vi "trig.vi"(8 "error in (no error)":errorcluster, 11 "p2p vst in":refnum<class "p2p vst.lvclass">) -> (0 "error out":errorcluster, 3 "p2p vst out":refnum<class "p2p vst.lvclass">)   [LabVIEW 2021, in "p2p vst.lvclass"]
uses:
  p2p vst.lvclass
  p2p vst.lvclass/p2p vst.ctl
  <instrlib>/niRFSG/niRFSG.llb/niRFSG Stream Endpoint Names.ctl
  <vilib>/FPGAPlugInAG/Dynamic/niLvFpga_P2PGetEndpoint_Dynamic.vi
  <vilib>/Utility/error.llb/Error Cluster From Error Code.vi
  <vilib>/rvi/errors/niLvFpgaAdjustHostInterfaceError.vi
  <vilib>/rvi/interface/nirviMethod/nirviMethod.xnode
  <vilib>/rvi/interface/nirviReadWriteControl/nirviReadWriteControl.xnode
  NiFpgaLv.dll
  <vilib>/rvi/interface/Simulation/niFpgaSimulationCallBeginRW.vi
  <vilib>/rvi/errors/niLvFpgaMergeErrorWithErrorCode.vi
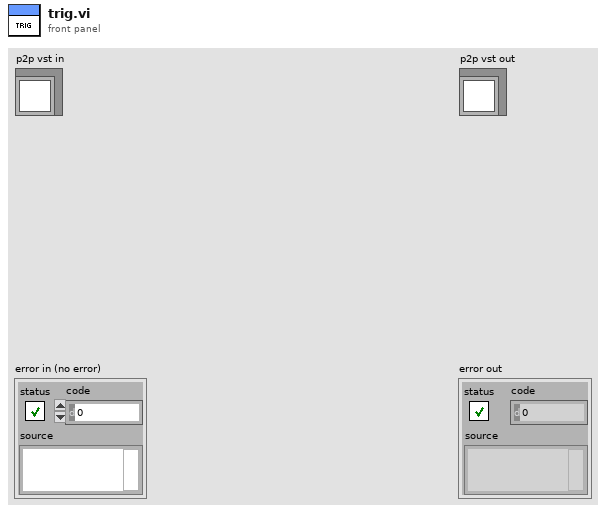
[diagram p1: front panel]
types:
  T1 = typedef "niRFSG Stream Endpoint Names.ctl" = string
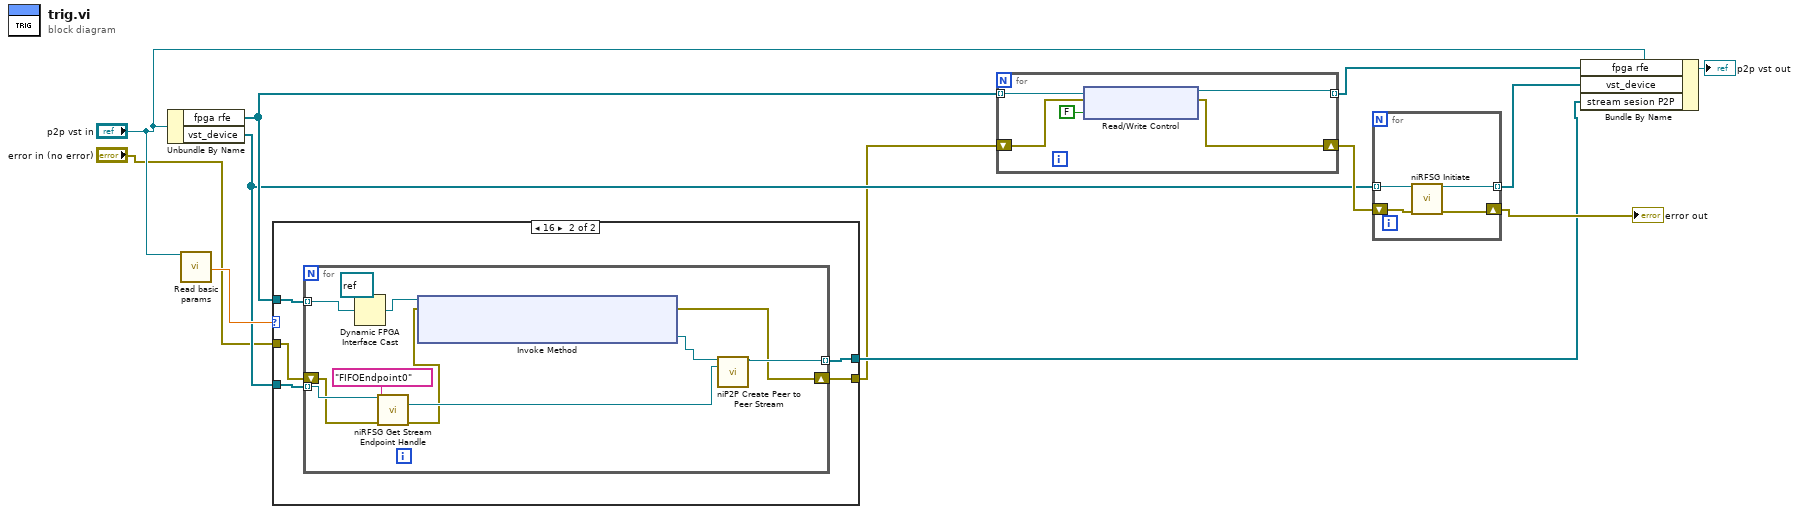
[diagram p0: block diagram]
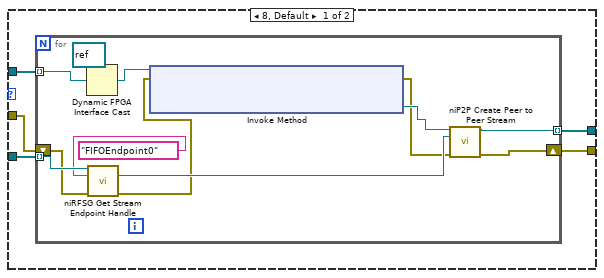
[diagram p2: hidden frame]
diagram:
  n1 = Unbundle By Name("p2p vst in") -> ("fpga rfe"=w5:refnum<k20>[], "vst_device"=w4:refnum<k15>[])
  n2 = call-dynamic "Read basic params.vi"("device_type in"="p2p vst in") -> ("SPC"=w6:dbl)  [unwired: 11 in, 7 out]
  n3 = case shown="16" w6 {
    tunnel: w5 -> [w17 w34]
    tunnel: w4 -> [w16 w33]
    tunnel: [w15 w32] -> w3
    tunnel: "error in (no error)" -> [w14 w31]
    tunnel: [w13 w30] -> w1
    frame 8, Default {
      n4 = for {
        tunnel: w17 -> [w25] mode=indexing
        tunnel: w16 -> [w29] mode=indexing
        tunnel: [w22] -> w15 mode=indexing
        shift-right: [w18] -> w13
        shift-left: w14 -> [w21]
        n5 = Dynamic FPGA Interface Cast(Session In=refnum<k20> refnum ("FPGA VI Reference Out"), Type=w25) -> (Session Out=w23:refnum<k20>)
        n6 = call <instrlib>:"niRFSG Get Stream Endpoint Handle.vi"("instrument handle"=w29, "stream endpoint"=T1 "FIFOEndpoint0", "error in"=w21) -> ("reader handle"=w27:refnum<k20>, "error out"=w20:errorcluster)  [unwired: 10 in, 1 out]
        n7 = xnode "Invoke Method"("FPGA VI Reference In"=w23, "error in"=w20) -> ("error out"=w19:errorcluster, "Writer"=w26:refnum<k20>)  [unwired: 1 out]
        n8 = call <vilib>:"niP2P Create Peer to Peer Stream.vi"("writer"=w26, "reader"=w27, "error in (no error)"=w19) -> ("stream session"=w22:refnum<k20>, "error out"=w18:errorcluster)  [unwired: 11 in]
      }
    }
    frame 16 {
      n9 = for {
        tunnel: w34 -> [w41] mode=indexing
        tunnel: w33 -> [w45] mode=indexing
        tunnel: [w38] -> w32 mode=indexing
        shift-right: [w35] -> w30
        shift-left: w31 -> [w37]
        n10 = Dynamic FPGA Interface Cast(Session In=refnum<k20> refnum ("FPGA VI Reference Out"), Type=w41) -> (Session Out=w39:refnum<k20>)
        n11 = call <instrlib>:"niRFSG Get Stream Endpoint Handle.vi"("instrument handle"=w45, "stream endpoint"=T1 "FIFOEndpoint0", "error in"=w37) -> ("reader handle"=w43:refnum<k20>, "error out"=w36:errorcluster)  [unwired: 10 in, 1 out]
        n12 = xnode "Invoke Method"("FPGA VI Reference In"=w39, "error in"=w36) -> ("error out"=w35:errorcluster, "Writer"=w42:refnum<k20>)  [unwired: 1 out]
        n13 = call <vilib>:"niP2P Create Peer to Peer Stream.vi"("writer"=w42, "reader"=w43) -> ("stream session"=w38:refnum<k20>)  [unwired: 12 in, 1 out]
      }
    }
  }
  n14 = for {
    tunnel: w5 -> [w50] mode=indexing
    tunnel: [w49] -> w11 mode=indexing
    shift-right: [w46] -> w12
    shift-left: w1 -> [w48]
    n15 = xnode "Read/Write Control"("FPGA VI Reference In"=w50, "error in"=w48, "reset system clock"=FALSE) -> ("FPGA VI Reference Out"=w49:refnum<k20>, "error out"=w46:errorcluster)
  }
  n16 = for {
    shift-right: [w52] -> w8
    shift-left: w12 -> [w53]
    tunnel: w4 -> [w54] mode=indexing
    tunnel: [w51] -> w9 mode=indexing
    n17 = call <instrlib>:"niRFSG Initiate.vi"("instrument handle"=w54, "error in"=w53) -> ("instrument handle out"=w51:refnum<k15>, "error out"=w52:errorcluster)  [unwired: 12 in]
  }
  "error out" <- w8
  n18 = Bundle By Name(cluster="p2p vst in", "fpga rfe"=w11, "vst_device"=w9, "stream sesion P2P"=w3) -> (→"p2p vst out":refnum<class "p2p vst.lvclass">)
